vi "encode.vi"(8 "error in (no error)":errorcluster caption="错误输入（无错误）", 11 "待发送数据":string[][](array[string])) -> (0 "error out":errorcluster caption="错误输出", 3 "通讯包字符串":string)   [LabVIEW 2016, in "数据传输系统-03.lvlib"]
panel:
  out "长度":i32
  # "AA720000000100020003000400053230313731323232303730353535"
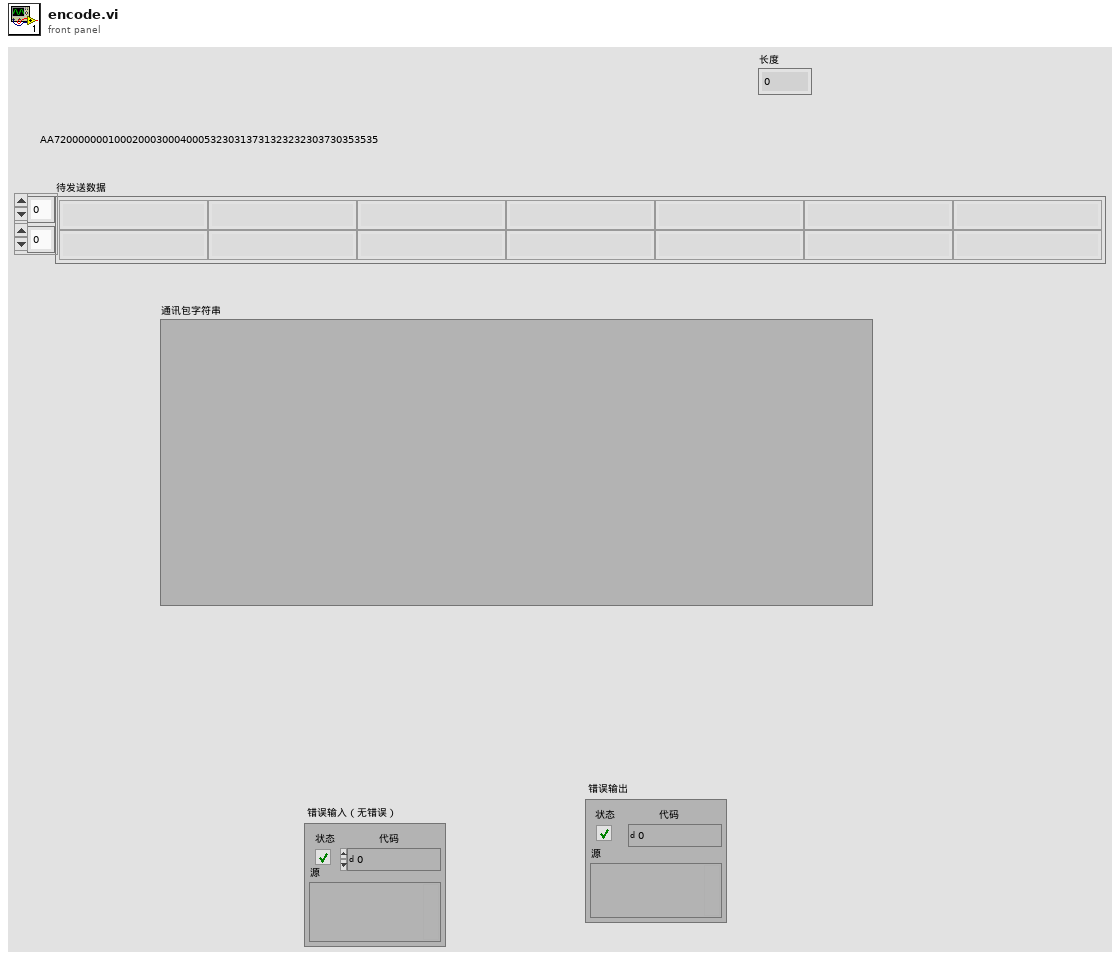
[diagram p1: front panel]
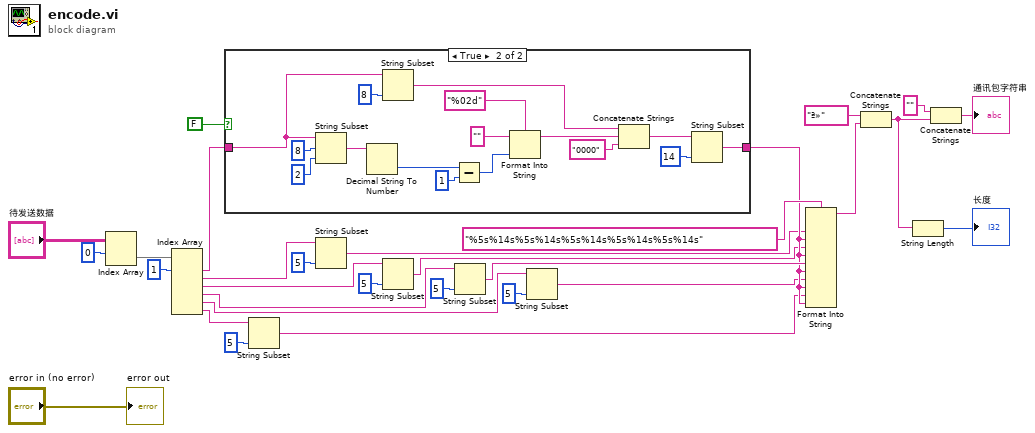
[diagram p0: block diagram]
diagram:
  n1 = Index Array(array="待发送数据", index (row)=0 ("索引 (行)")) -> (element=w27:string[])  [unwired: 1 in]
  n2 = Index Array(array=w27, index #1=1 ("索引")) -> (element #1=w5:string, element #2=w11:string, element #3=w9:string, element #4=w18:string, element #5=w3:string, element #6=w6:string)  [unwired: 5 in]
  n3 = case shown="True" FALSE {
    tunnel: [w31 w46] -> w15
    tunnel: w5 -> [w31 w32]
    frame False {
    }
    frame True {
      n4 = String Subset(string=w32, offset (0)=8 ("偏移量(0)"), length (rest)=2 ("长度（剩余）")) -> (substring=w42:string)
      n5 = Decimal String To Number(string=w42) -> (number=w40:i32)  [unwired: 2 in, 1 out]
      n6 = String Subset(string=w32, length (rest)=8 ("长度（剩余）")) -> (substring=w36:string)  [unwired: 1 in]
      n7 = Subtract(x=w40, y=1) -> (x-y=w37:i32)
      n8 = Format Into String(format string="%02d" ("格式字符串"), initial string="" ("初始字符串"), w37) -> (resulting string=w35:string)  [unwired: 1 in, 1 out]
      n9 = Concatenate Strings(w36, w35, "0000" ("字符串")) -> (w34:string)
      n10 = String Subset(string=w34, length (rest)=14 ("长度（剩余）")) -> (substring=w46:string)  [unwired: 1 in]
    }
  }
  n11 = String Subset(string=w6, length (rest)=5 ("长度（剩余）")) -> (substring=w7:string)  [unwired: 1 in]
  n12 = String Subset(string=w11, length (rest)=5 ("长度（剩余）")) -> (substring=w10:string)  [unwired: 1 in]
  n13 = String Subset(string=w9, length (rest)=5 ("长度（剩余）")) -> (substring=w8:string)  [unwired: 1 in]
  n14 = String Subset(string=w18, length (rest)=5 ("长度（剩余）")) -> (substring=w16:string)  [unwired: 1 in]
  n15 = String Subset(string=w3, length (rest)=5 ("长度（剩余）")) -> (substring=w1:string)  [unwired: 1 in]
  n16 = Format Into String(format string="%5s%14s%5s%14s%5s%14s%5s%14s%5s%14s" ("格式字符串"), w10, w15, w8, w15, w16, w15, w1, w15, w7, w15) -> (resulting string=w19:string)  [unwired: 2 in, 1 out]
  n17 = Concatenate Strings("ª»", w19) -> (w22:string)
  n18 = String Length(string=w22) -> (length=→"长度":i32)
  n19 = Concatenate Strings("", w22) -> (→"通讯包字符串":string)
  "error out" <- "error in (no error)"
